vi "close.vi"(8 "error in":errorcluster, 11 "UI Reference runtime in":refnum<class "io runtime.lvclass">) -> (0 "error out":errorcluster)   [LabVIEW 2015, in "io runtime.lvclass"]
doc: "Provides an interface for terminating a module instance. While this interface performs no operations, a child should close and deallocate any open references or memory."
uses:
  io runtime.lvclass
  io runtime.lvclass/io runtime.ctl
  <vilib>/Utility/error.llb/Error Cluster From Error Code.vi
  <vilib>/FPGAPlugInAG/Dynamic/niLvFpga_Close_Dynamic.vi
  <vilib>/rvi/interface/nirviMethod/nirviMethod.xnode
  <vilib>/rvi/interface/nirviCloseFPGA/nirviCloseFPGA.xnode
  <vilib>/FPGAPlugInAG/Dynamic/niLvFpga_StopFifo_Dynamic.vi
  <vilib>/rvi/errors/niLvFpgaMergeErrorWithErrorCode.vi
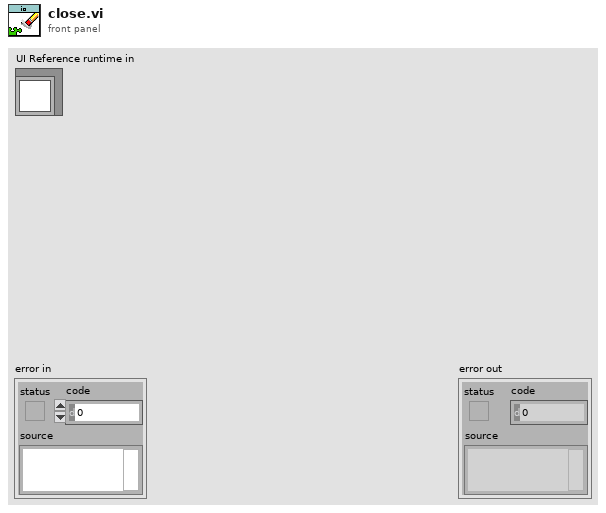
[diagram p1: front panel]
types:
  T1 = typedef "io runtime.lvclass/control index set.ctl" = cluster{"data type":T2, "fpga res type":T3[], "fpga resource":refnum<k20>[], "data indexes":i32[], "fifo timeout":refnum<k20>[], "fifo reset":refnum<k20>[], "fifo average":i32[], "fifo samples":u32[], "fifo channels":u32[]}
  T2 = typedef "tag bus.lvlib/tag descriptor.lvclass/Data Type.ctl" = enum16{"Double", "Single", "I64", "I32", "I16", "I8", "U64", "U32", "U16", "U8", "Boolean", "String", "Array of Double", "Array of Single", "Array of I64", "Array of I32", "Array of I16", "Array of I8", "Array of U64", "Array of U32", "Array of U16", "Array of U8", "Array of Boolean", "Array of String"}
  T3 = typedef "io configuration.lvclass/fpga resource supported data types.ctl" = enum16{"Invalid Type", "Single", "I64", "I32", "I16", "I8", "U64", "U32", "U16", "U8", "Boolean", "FXP I,20,5", "FXP I,24,5", "FXP I,24,10", "Fifo 1023,I16"}
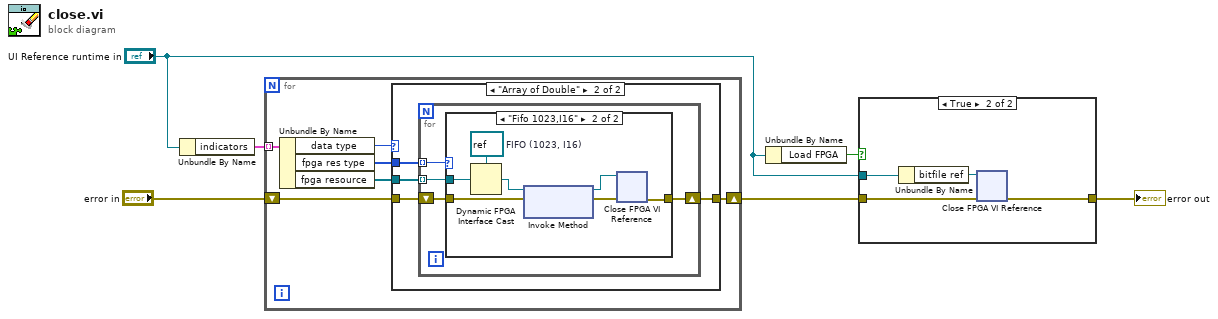
[diagram p0: block diagram]
diagram:
  n1 = Unbundle By Name("UI Reference runtime in") -> ("indicators"=w3:T1[])
  n2 = for {
    tunnel: w3 -> [w12] mode=indexing
    shift-right: [w7] -> w1
    shift-left: "error in" -> [w8]
    n3 = Unbundle By Name(w12) -> ("data type"=w11:T2, "fpga res type"=w10:T3[], "fpga resource"=w9:refnum<k20>[])
    n4 = case shown="\"Array of Double\"" w11 {
      tunnel: w10 -> [_ w17]
      tunnel: w9 -> [_ w16]
      tunnel: w8 -> [w13 w15]
      tunnel: [w13 w14] -> w7
      frame Default {
      }
      frame "Array of Double" {
        n5 = for {
          tunnel: w17 -> [w21] mode=indexing
          tunnel: w16 -> [w20] mode=indexing
          shift-right: [w18] -> w14
          shift-left: w15 -> [w19]
          n6 = case shown="\"Fifo 1023,I16\"" w21 {
            tunnel: w20 -> [_ w28]
            tunnel: w19 -> [w22 w29]
            tunnel: [w22 w24] -> w18
            frame Default {
            }
            frame "Fifo 1023,I16" {
              w27 = refnum<k20> refnum  # FIFO (1023, I16)
              n7 = Dynamic FPGA Interface Cast(Session In=w27, Type=w28) -> (Session Out=w26:refnum<k20>)
              n8 = xnode "Invoke Method"("FPGA VI Reference In"=w26, "error in"=w29) -> ("FPGA VI Reference Out"=w23:refnum<k20>, "error out"=w25:errorcluster)
              n9 = xnode "Close FPGA VI Reference"("FPGA VI Reference In"=w23, "error in"=w25) -> ("error out"=w24:errorcluster)
            }
          }
        }
      }
    }
  }
  n10 = Unbundle By Name("UI Reference runtime in") -> ("Load FPGA"=w5:bool)
  n11 = case shown="True" w5 {
    tunnel: w1 -> [w30 w34]
    tunnel: [w30 w33] -> w6
    tunnel: "UI Reference runtime in" -> [_ w32]
    frame False {
    }
    frame True {
      n12 = Unbundle By Name(w32) -> ("bitfile ref"=w31:refnum<k20>)
      n13 = xnode "Close FPGA VI Reference"("FPGA VI Reference In"=w31, "error in"=w34) -> ("error out"=w33:errorcluster)
    }
  }
  "error out" <- w6
